vi "_Read.vi"(8 "error in (no error)":errorcluster, 11 "Power Meter in":refnum<class "Power Meter.lvclass">) -> (0 "error out":errorcluster, 2 "X array":T1, 3 "Power Meter out":refnum<class "Power Meter.lvclass">)   [LabVIEW 2012, in "Power Meter.lvclass"]
doc: "(Protected, Dynamic, Pure Virtual/Abstract) Perform a measurement and return one or more channels of data. Outsiders should not call this method, but instead the public \"Read Power.vi\".\n\nThis vi compares the current point to the previous and returns 0 if current if more than twice as much as previous. It also creates a warning, error value of 1."
uses:
  Power Meter.lvclass
  Utility Classes/Readable/X array.ctl
  Utility Classes/Readable/X.ctl
  Utility Classes/Readable/Readable.lvclass
  Power Meter.lvclass/Power Meter.ctl
  Newport 1830-C/Newport 1830-C.lvlib
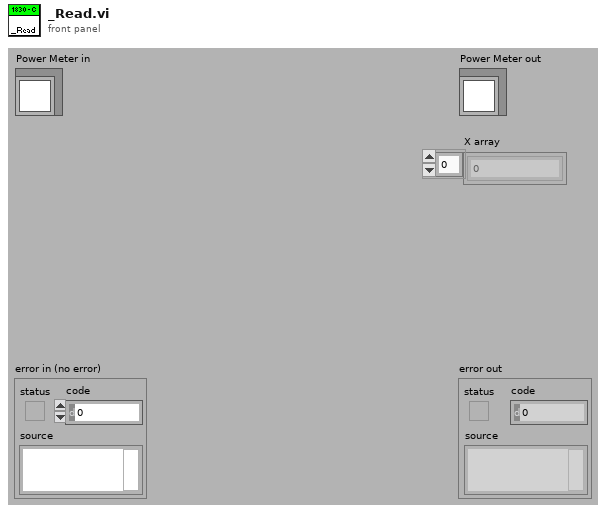
[diagram p1: front panel]
types:
  T1 = typedef "Readable.lvclass/X array.ctl" = T2[]
  T2 = typedef "Readable.lvclass/X.ctl" = dbl
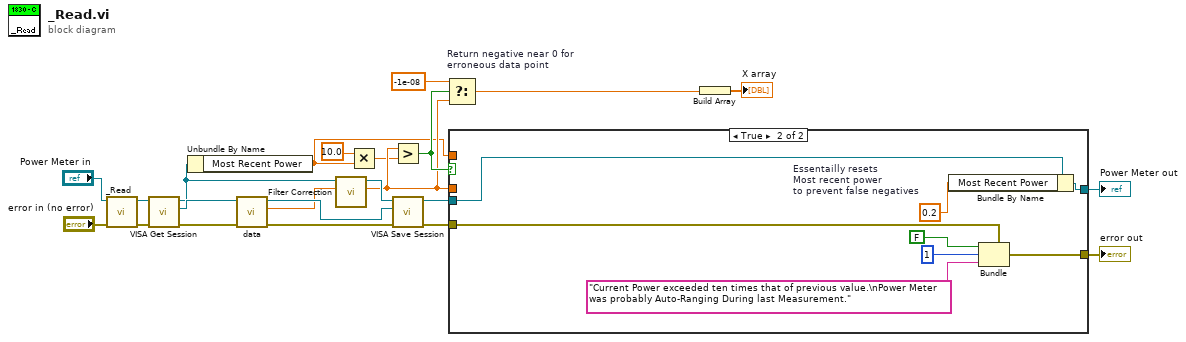
[diagram p0: block diagram]
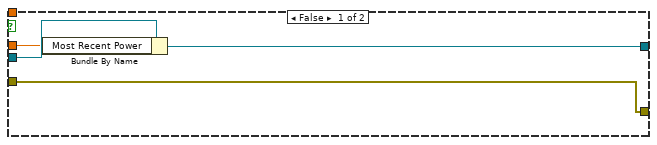
[diagram p2: hidden frame]
diagram:
  n1 = call-parent "_Read.vi"("error in (no error)"="error in (no error)", "Readable in"="Power Meter in") -> ("error out"=w17:errorcluster, "Readable out"=w21:refnum<class "Power Meter.lvclass">)  [unwired: 7 in, 1 out]
  n2 = call-dynamic "VISA Get Session.vi"("error in (no error)"=w17, "Instrument.lvclass in"=w21) -> ("error out"=w18:errorcluster, "VISA Resource Name"=w20:refnum<visa-resource-name>, "Instrument.lvclass out"=w5:refnum<class "Power Meter.lvclass">)  [unwired: 7 out]
  n3 = Unbundle By Name(w5) -> ("Most Recent Power"=w1:dbl)
  n4 = call "data.vi"("error in (no error)"=w18, "VISA resource name"=w20) -> ("error out"=w8:errorcluster, "Power"=w6:dbl, "VISA resource name out"=w16:refnum<visa-resource-name>)  [unwired: 7 in]
  n5 = call "Filter Correction.vi"("Read Power"=w6, "Power Meter.lvclass In"=w5) -> ("Corrected Power"=w4:dbl, "Power Meter.lvclass Out"=w7:refnum<class "Power Meter.lvclass">)  [unwired: 8 in]
  n6 = Multiply(x=10.0, y=w1) -> (x*y=w2:dbl)
  n7 = Greater?(x=w4, y=w2) -> (0:w14:bool)
  n8 = call-dynamic "VISA Save Session.vi"("error in (no error)"=w8, "VISA Resource Name"=w16, "Instrument.lvclass in"=w7) -> ("error out"=w13:errorcluster, "Instrument.lvclass out"=w11:refnum<class "Power Meter.lvclass">)  [unwired: 7 out]
  n9 = Select "Return negative near 0 for\nerroneous data point"(t=-1e-08, s=w14, f=w4) -> (s? t:f=w10:dbl)
  n10 = case shown="True" w14 {
    tunnel: w13 -> [w27 w35]
    tunnel: [w27 w31] -> w12
    tunnel: w11 -> [w26 w30]
    tunnel: w4 -> [w24 _]
    tunnel: [w25 w29] -> w9
    tunnel: w1 -> [_ _]
    frame False {
      n11 = Bundle By Name(cluster=w26, "Most Recent Power"=w24) -> (w25:refnum<class "Power Meter.lvclass">)
    }
    frame True {
      w28 = 0.2  # Essentailly resets Most recent power to prevent false negatives
      n12 = Bundle By Name(cluster=w30, "Most Recent Power"=w28) -> (w29:refnum<class "Power Meter.lvclass">)
      n13 = Bundle(cluster=w35, "status"=FALSE, "code"=1, "source"="Current Power exceeded ten times that of previous value.\nPower Meter was probably Auto-Ranging During last Measurement.") -> (w31:errorcluster)
    }
  }
  "error out" <- w12
  "Power Meter out" <- w9
  n14 = Build Array(w10) -> (→"X array":dbl[])
